vi "LVFunction_Imop_Compute_WavefrontFromCoef.vi"(0 "Phase":refnum<class "Phase.lvclass">, 5 "ComputePhaseSet":refnum<class "ComputePhaseSet.lvclass">, 7 "ModalCoef":refnum<class "ModalCoef.lvclass">, 11 "error IO":errorcluster) -> (4 "Phase":refnum<class "Phase.lvclass">, 6 "ComputePhaseSet (dup)":refnum<class "ComputePhaseSet.lvclass">, 8 "ModalCoef (dup)":refnum<class "ModalCoef.lvclass">, 15 "error IO out":errorcluster)   [LabVIEW 2020]
doc: "Compute phase from modal coefficients in a given basis of polynomials provided\nby ComputePhaseSet.\n\n<B>ComputePhaseSetIn</B> : ComputePhaseSet object.\n<B>ComputePhaseSetOut</B> : ComputePhaseSet object.\n<B>ModalCoeffs</B> : ModalCoef object.\n<B>Phase</B> : phase object. Phase values are expressed in um. Phase size and steps are set from ModalCoef object (Pupil object size)."
uses:
  ModalCoef.lvclass
  ComputePhaseSet.lvclass
  Phase.lvclass
  LVClass_ComputePhaseSet Read ComputePhaseSet.vi
  LVClass_ModalCoef Read ModalCoef.vi
  LVClasse_Phase Read SurfaceFloatWithPupil.vi
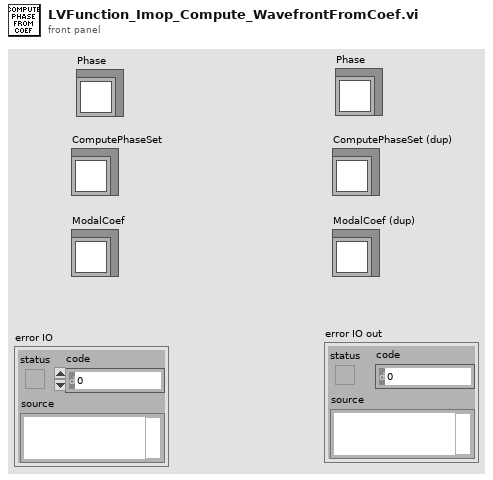
[diagram p1: front panel]
types:
  T1 = typedef "ClassID.ctl" = i64
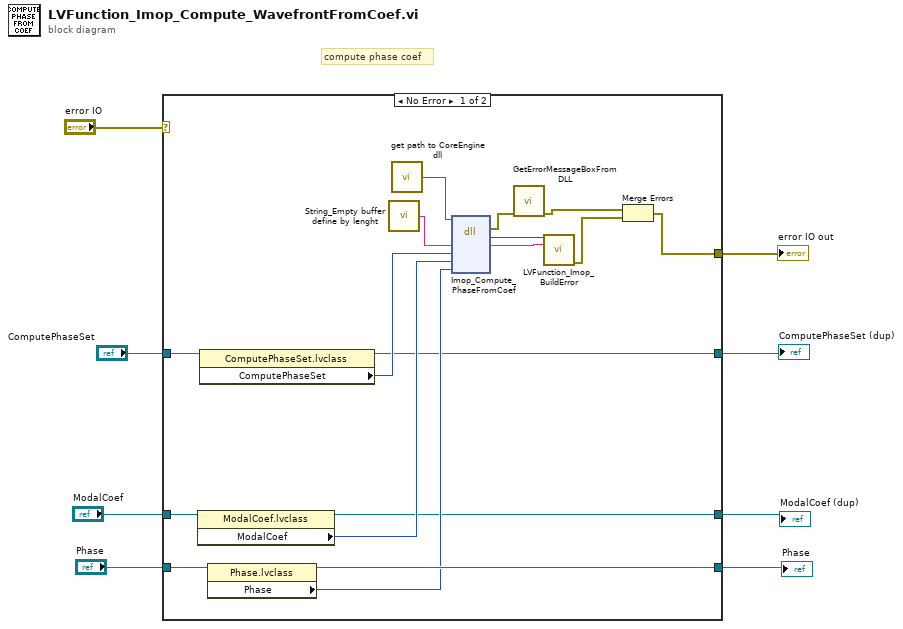
[diagram p0: block diagram]
diagram:
  # "compute phase coef"
  n1 = case shown="No Error" "error IO" {
    selector: "error IO" -> [_ w29]
    tunnel: [w10 w29] -> w7
    tunnel: [w20 w28] -> w2
    tunnel: "Phase" -> [w19 w28]
    tunnel: "ModalCoef" -> [w18 w27]
    tunnel: "ComputePhaseSet" -> [w17 w26]
    tunnel: [w13 w27] -> w5
    tunnel: [w9 w26] -> w1
    frame No Error {
      n2 = property class="ModalCoef.lvclass"(reference=w18) -> (reference out=w13:refnum<class "ModalCoef.lvclass">, "ModalCoef"=w15:T1)  [unwired: 1 in, 1 out]
      n3 = property class="ComputePhaseSet.lvclass"(reference=w17) -> (reference out=w9:refnum<class "ComputePhaseSet.lvclass">, "ComputePhaseSet"=w16:T1)  [unwired: 1 in, 1 out]
      n4 = property class="Phase.lvclass"(reference=w19) -> (reference out=w20:refnum<class "Phase.lvclass">, "Phase"=w14:T1)  [unwired: 1 in, 1 out]
      n5 = call "String_Empty buffer define by lenght.vi"() -> ("Empty buffer"=w23:string)  [unwired: 1 in]
      n6 = call "get path to CoreEngine dll.vi"() -> ("path to wavekit library"=w22:path)  [unwired: 14 in, 1 out]
      n7 = dll-call lib="D:/FLE/0.Code/CoreEngine4_Suite/LV2011_interface/DLLs/c_interface_vc100.dll" fn="Imop_Compute_PhaseFromCoef"(path in=w22, "message"=w23, "ComputePhaseSet"=w16, "Modalcoefs"=w15, "phase"=w14) -> (error out=w21:errorcluster, "return type"=w25:i32, "message"=w24:string)  [unwired: 5 in, 1 out]
      n8 = call "GetErrorMessageBoxFromDLL.vi"("error IN"=w21) -> ("error OUT"=w12:errorcluster)  [unwired: 10 in]
      n9 = call "LVFunction_Imop_BuildError.vi"("code"=w25, "String to Prepend to source (\"\")"=w24) -> ("error out"=w11:errorcluster)  [unwired: 13 in]
      n10 = Merge Errors(w12, w11) -> (w10:errorcluster)
    }
    frame Error {
    }
  }
  "error IO out" <- w7
  "ModalCoef (dup)" <- w5
  "ComputePhaseSet (dup)" <- w1
  "Phase" <- w2
